vi "zern2command_test.vi"(7 "Initial haso file":path=path "D:/SystemAlignment/system_aberration_residual_20191015.has", 8 "error in (no error)":errorcluster, 9 "interaction matrix file":path=path "D:/YD/data/20191206/im.aomi", 10 "Zern coef in":sgl[](array[numeric]), 11 "Zern index in":i32[](array[numeric])) -> (0 "error out":errorcluster, 2 "Zern coef out":sgl[](array[numeric]), 3 "Offset positions":sgl[](graph))   [LabVIEW 2018]
uses:
  <userlib>/WaveKit.lib/Classes/ModalCoef/ModalCoef.lvclass
  <userlib>/WaveKit.lib/Controls/Pupil.lvclass
panel:
  out "Number of Coefficients":i32
  out "Zern index out":i32[](array[numeric])
  in  "Output folder":path=path "D:/Data/20200122_Test"
  in  "Output file name":string="test_zern2command.dat"
  in  "Hasao configuration file":path=path "C:/Program Files (x86)/Imagine Optic/Configuration Files/HASO3_first_7364.dat"
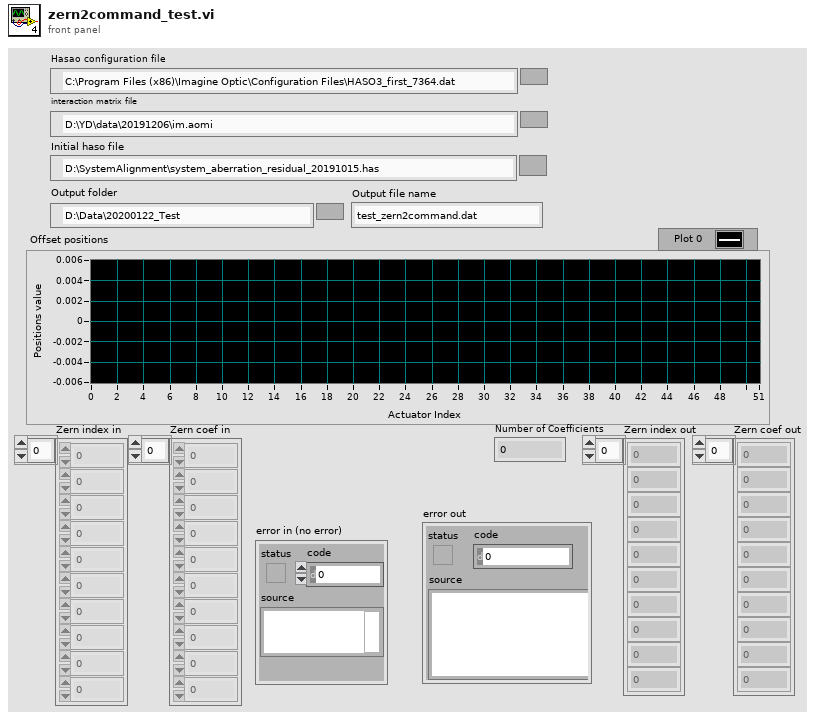
[diagram p1: front panel]
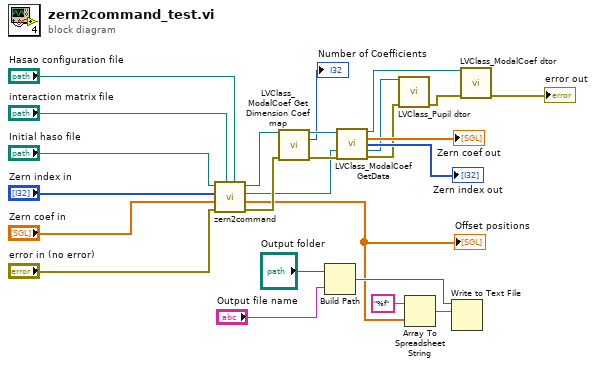
[diagram p0: block diagram]
diagram:
  n1 = call "zern2command.vi"("Hasao configuration file"="Hasao configuration file", "interaction matrix file"="interaction matrix file", "error in (no error)"="error in (no error)", "Zern coef in"="Zern coef in", "Zern index in"="Zern index in", "Initial haso file"="Initial haso file") -> ("error out"=w11:errorcluster, "Offset Positions"=w2:sgl[], "Zern pupil out"=w1:refnum<class "Pupil.lvclass">, "ModalCoef out"=w12:refnum<class "ModalCoef.lvclass">)  [unwired: 2 in]
  "Offset positions" <- w2
  n2 = call <userlib>:"LVClass_ModalCoef Get Dimension Coef map.vi"("ModalCoef in"=w12, "error in (no error)"=w11) -> ("ModalCoef out"=w15:refnum<class "ModalCoef.lvclass">, "# of coef"=→"Number of Coefficients":i32, "error out"=w10:errorcluster)  [unwired: 11 in]
  n3 = Build Path(base path="Output folder", name or relative path="Output file name") -> (appended path=w17:path)
  n4 = call <userlib>:"LVClass_ModalCoef GetData.vi"("ModalCoef in"=w15, "Pupil.lvclass"=w1, "error in (no error)"=w10) -> ("ModalCoef out"=w13:refnum<class "ModalCoef.lvclass">, "coef"=→"Zern coef out":sgl[], "index"=→"Zern index out":u32[], "Pupil.lvclass (dup)"=w7:refnum<class "Pupil.lvclass">, "error out"=w6:errorcluster)  [unwired: 8 in]
  n5 = call <userlib>:"LVClass_Pupil dtor.vi"("Pupil in"=w7, "error in (no error)"=w6) -> ("error out"=w5:errorcluster)  [unwired: 12 in, 1 out]
  n6 = Array To Spreadsheet String(array=w2, 3:"%f") -> (spreadsheet string=w20:string)  [unwired: 1 in]
  n7 = Write to Text File(file (use dialog)=w17, text=w20) -> ()  [unwired: 2 in, 3 out]
  n8 = call <userlib>:"LVClass_ModalCoef dtor.vi"("ModalCoef in"=w13, "error in (no error)"=w5) -> ("error out"=→"error out":errorcluster)  [unwired: 12 in, 1 out]
